vi "Separate Selected Layers.vi"(7 "Active Indices":i32[](array[numeric]), 11 "All Layers":refnum<class "Layer.lvclass">[](array[class])) -> (1 "Layers out in Array":refnum<class "Layer.lvclass">[](array[class]), 3 "Layers out not in Array":refnum<class "Layer.lvclass">[](array[class]))   [LabVIEW 2021]
uses:
  vi.lib/LabVIEW Icon API/lv_icon/Classes/Layer/Layer.lvclass
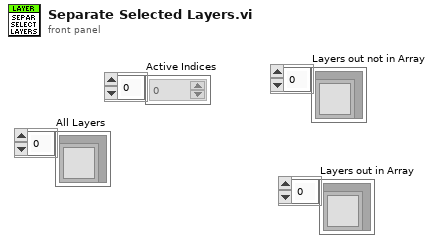
[diagram p1: front panel]
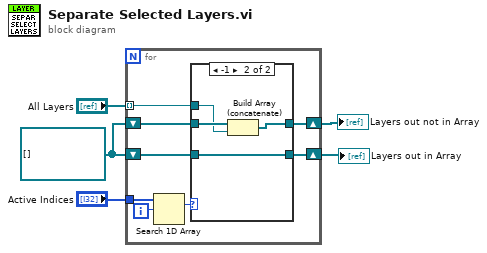
[diagram p0: block diagram]
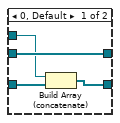
[diagram p2: hidden frame]
diagram:
  w1 = refnum<class "Layer.lvclass">[] []
  n1 = for {
    tunnel: "Active Indices" -> [w13]
    tunnel: "All Layers" -> [w10] mode=indexing
    shift-right: [w6] -> w2
    shift-left: w1 -> [w7]
    shift-right: [w8] -> w3
    shift-left: w1 -> [w9]
    i -> [w12]
    n2 = Search 1D Array(1D array=w13, element=w12) -> (index of element=w11:i32)  [unwired: 1 out]
    n3 = case shown="-1" w11 {
      tunnel: w10 -> [w15 w20]
      tunnel: w9 -> [w17 w21]
      tunnel: [w17 w19] -> w8
      tunnel: w7 -> [w16 w18]
      tunnel: [w14 w18] -> w6
      frame 0, Default {
        n4 = Build Array (concatenate)(w15, w16) -> (w14:refnum<class "Layer.lvclass">[])
      }
      frame -1 {
        n5 = Build Array (concatenate)(w21, w20) -> (w19:refnum<class "Layer.lvclass">[])
      }
    }
  }
  "Layers out not in Array" <- w3
  "Layers out in Array" <- w2
